vi "DequeueExperiment.vi"(0 "object in":refnum<class "Experiment.lvclass">, 5 "error in (no error)":errorcluster) -> (14 "object out":refnum<class "Experiment.lvclass">, 15 "Message":string, 16 "Message Data":variant, 17 "QueueEmpty":bool, 19 "error out":errorcluster)   [LabVIEW 2019, in "Experiment.lvclass"]
uses:
  Experiment.lvclass
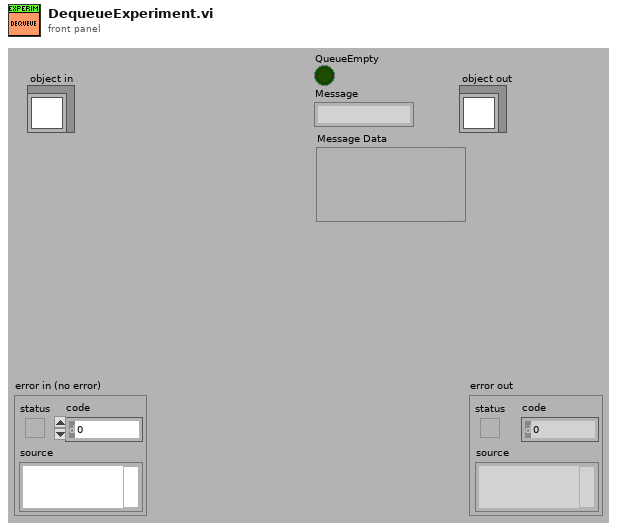
[diagram p1: front panel]
types:
  T1 = cluster{"Message":string, "Message Data":variant}
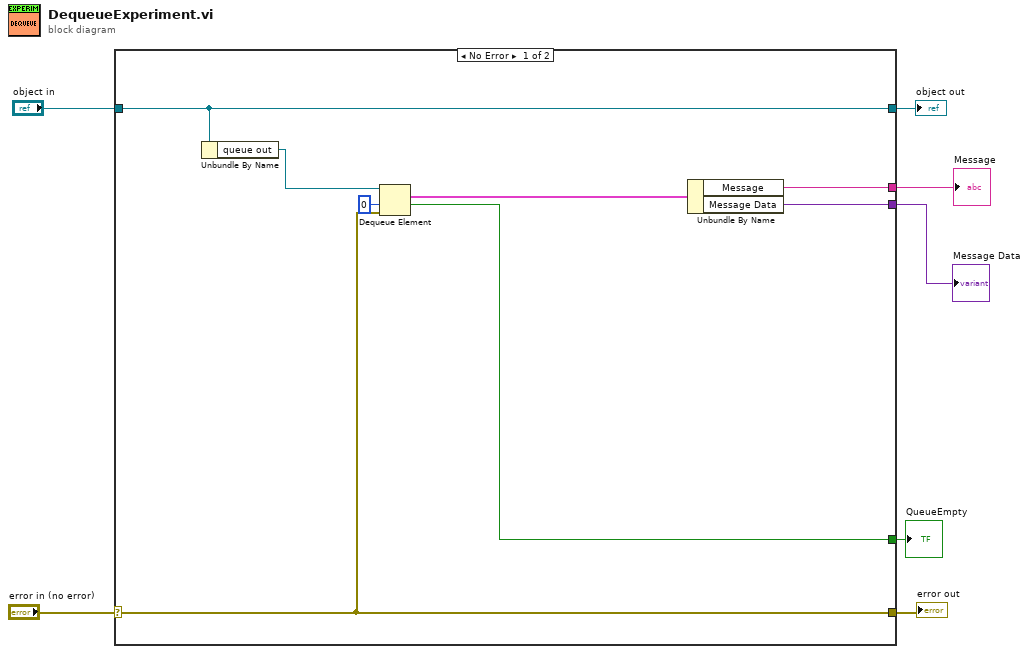
[diagram p0: block diagram]
diagram:
  n1 = case shown="No Error" "error in (no error)" {
    selector: "error in (no error)" -> [w13 w17]
    tunnel: [w13 w17] -> w6
    tunnel: [w15 w16] -> w4
    tunnel: "object in" -> [w15 w16]
    tunnel: [w11 _] -> w3
    tunnel: [w9 _] -> w2
    tunnel: [w8 _] -> w1
    frame No Error {
      n2 = Unbundle By Name(w15) -> ("queue out"=w14:refnum<queue>)
      n3 = Dequeue Element(queue=w14, timeout in ms (-1)=0, error in (no error)=w13) -> (element=w10:T1, timed out?=w11:bool)  [unwired: 2 out]
      n4 = Unbundle By Name(w10) -> ("Message"=w9:string, "Message Data"=w8:variant)
    }
    frame Error {
    }
  }
  "error out" <- w6
  "object out" <- w4
  "QueueEmpty" <- w3
  "Message" <- w2
  "Message Data" <- w1
